vi "写入配置文件引用.vi"(8 "error in (no error)":errorcluster caption="错误输入（无错误）", 10 "config data":T1 caption="配置数据", 11 "启动器输入":refnum<class "启动器.lvclass">) -> (0 "error out":errorcluster caption="错误输出", 3 "启动器输出":refnum<class "启动器.lvclass">)   [LabVIEW 2017, in "启动器.lvlib" / "启动器.lvclass"]
uses:
  <vilib>/Utility/config.llb/Config Data RefNum.ctl
  <vilib>/Utility/config.llb/NI_LVConfig.lvlib
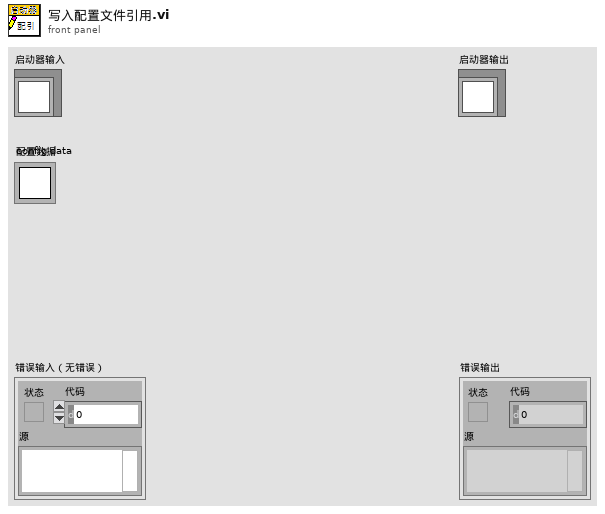
[diagram p1: front panel]
types:
  T1 = typedef "NI_LVConfig.lvlib/Config Data RefNum.ctl" = refnum<k1>
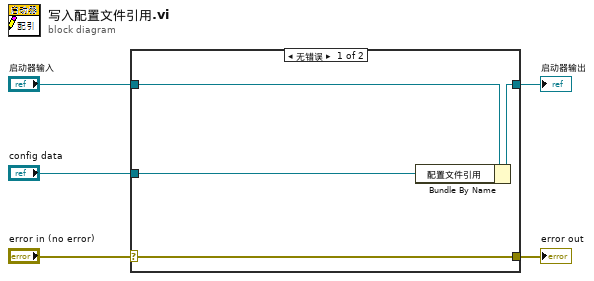
[diagram p0: block diagram]
diagram:
  n1 = case shown="无错误" "error in (no error)" {
    selector: "error in (no error)" -> [w9 w10]
    tunnel: [w9 w10] -> w4
    tunnel: [w7 w11] -> w2
    tunnel: "启动器输入" -> [w8 w11]
    tunnel: "config data" -> [w6 _]
    frame No Error {
      n2 = Bundle By Name(cluster=w8, "配置文件引用"=w6) -> (w7:refnum<class "启动器.lvclass">)
    }
    frame Error {
    }
  }
  "error out" <- w4
  "启动器输出" <- w2
